vi "VIQA VI Info Set.vi"(4 "Icon":refnum<class "Icon.lvclass">, 6 "NewIcon":bool, 8 "error in (no error)":errorcluster, 9 "NewLegal":string, 10 "NewDesc":string, 11 "VI Refnum":refnum<vi>) -> (0 "error out":errorcluster, 3 "dup VI Refnum":refnum<vi>)   [LabVIEW 2018, in "VI Quality.lvlib"]
doc: "This updates and saves the VI with the new information."
uses:
  VI Quality.lvlib
  <vilib>/LabVIEW Icon API/LabVIEW Icon API.lvlib
  <vilib>/LabVIEW Icon API/lv_icon/Classes/Icon/Icon.lvclass
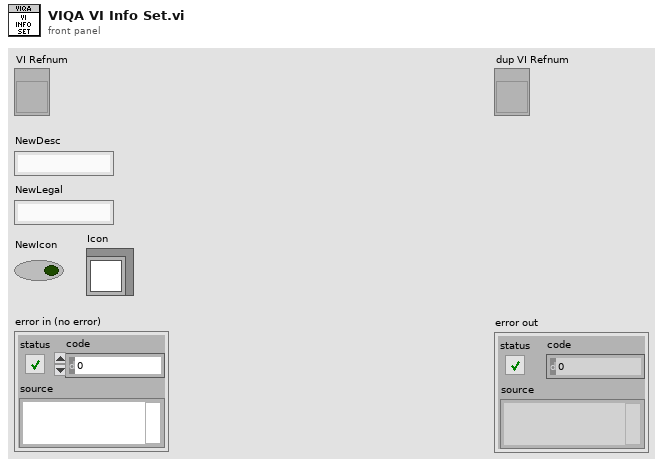
[diagram p1: front panel]
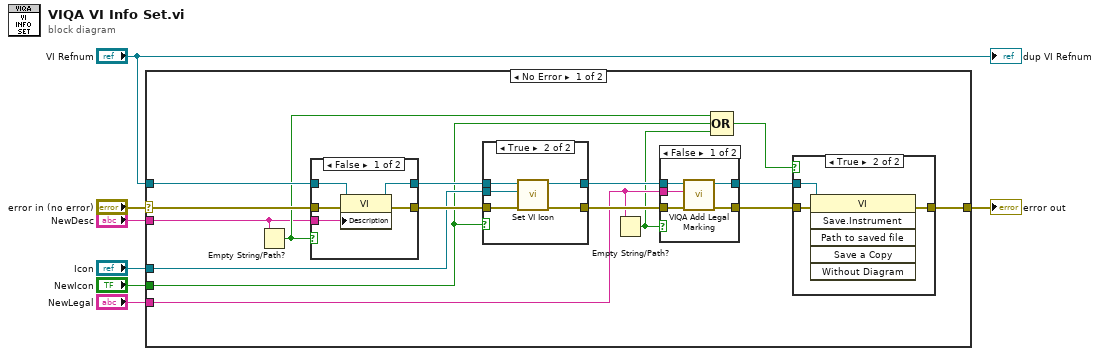
[diagram p0: block diagram]
diagram:
  n1 = case shown="No Error" "error in (no error)" {
    selector: "error in (no error)" -> [w23 w49]
    tunnel: "VI Refnum" -> [w22 _]
    tunnel: [w19 w49] -> w6
    tunnel: "NewDesc" -> [w12 _]
    tunnel: "Icon" -> [w11 _]
    tunnel: "NewIcon" -> [w9 _]
    tunnel: "NewLegal" -> [w10 _]
    frame No Error {
      n2 = Empty String/Path?(string/path=w12) -> (empty?=w13:bool)
      n3 = case shown="False" w13 {
        tunnel: w23 -> [w46 w48]
        tunnel: w22 -> [w45 w47]
        tunnel: [w44 w48] -> w21
        tunnel: [w43 w47] -> w20
        tunnel: w12 -> [w42 _]
        frame False {
          n4 = property class="VI"(reference=w45, error in=w46, "Description"=w42) -> (reference out=w43:refnum<vi>, error out=w44:errorcluster)
        }
        frame True {
        }
      }
      n5 = case shown="True" w9 {
        tunnel: w21 -> [w35 w41]
        tunnel: w20 -> [w36 w40]
        tunnel: [w35 w39] -> w16
        tunnel: [w36 w38] -> w14
        tunnel: w11 -> [_ w37]
        frame False {
        }
        frame True {
          n6 = call <vilib>:"Set VI Icon.vi"("error in (no error)"=w41, "Icon"=w37, "VI Refnum in"=w40) -> ("error out"=w39:errorcluster, "VI Refnum out"=w38:refnum<vi>)  [unwired: 7 in]
        }
      }
      n7 = Empty String/Path?(string/path=w10) -> (empty?=w8:bool)
      n8 = case shown="False" w8 {
        tunnel: [w28 w29] -> w17
        tunnel: w16 -> [w27 w29]
        tunnel: [w26 w30] -> w15
        tunnel: w14 -> [w25 w30]
        tunnel: w10 -> [w24 _]
        frame False {
          n9 = call "VIQA Add Legal Marking.vi"("error in (no error)"=w27, "Legal Marking"=w24, "VI Refnum"=w25) -> ("error out"=w28:errorcluster, "dup VI Refnum"=w26:refnum<vi>)  [unwired: 7 in]
        }
        frame True {
        }
      }
      n10 = Compound Arithmetic op=OR(w13, w9, w8) -> (w18:bool)
      n11 = case shown="True" w18 {
        tunnel: w17 -> [w31 w34]
        tunnel: [w31 w33] -> w19
        tunnel: w15 -> [_ w32]
        frame False {
        }
        frame True {
          n12 = invoke class="VI" method="Save.Instrument"(reference=w32, error in=w34) -> (error out=w33:errorcluster)  [unwired: 4 in, 5 out]
        }
      }
    }
    frame Error {
    }
  }
  "error out" <- w6
  "dup VI Refnum" <- "VI Refnum"
